vi "BRig_RT__Case_Exp__storeData__endExp__v2.vi"(0 "input_dataBlock":u16[][](array[numeric]), 1 "input_dataCurrent":u16[](array[numeric]), 2 "input_dataLick":u16[][](array[numeric]), 3 "input_dataLC":u16[](array[numeric]), 4 "input_dataExp":u16[](array[numeric]), 5 "input_dataTrial":u16[][](array[numeric]), 7 "input_dataExp_end":u16[](array[numeric]), 9 "input_dataLC_end":u16[](array[numeric]), 11 "input_dataMTrig":u16[](array[numeric]), 12 "input_dataAnalog":u16[][](array[numeric]), 13 "input_dataAnalog_length":i32) -> ()   [LabVIEW 2014]
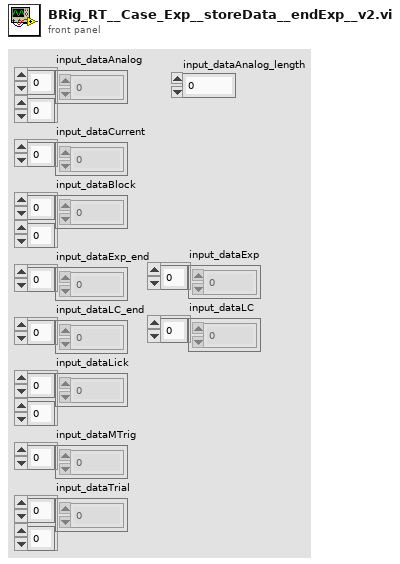
[diagram p1: front panel]
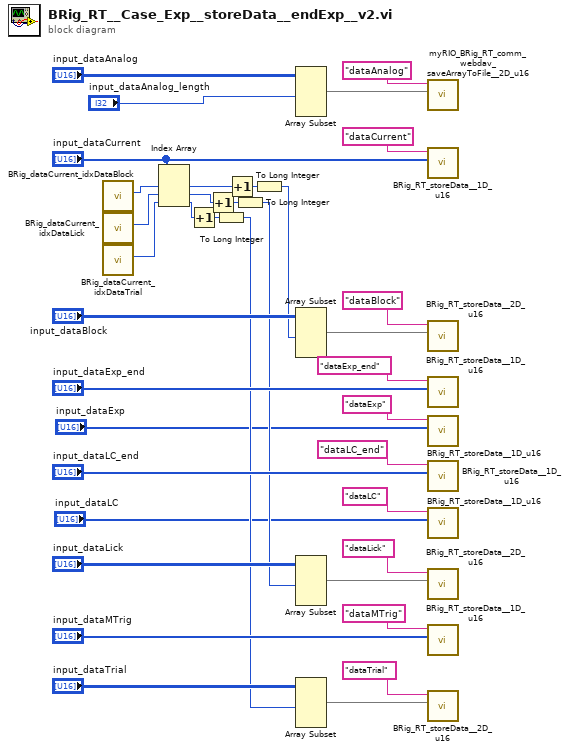
[diagram p0: block diagram]
diagram:
  n1 = call "BRig_dataCurrent_idxDataBlock.vi"() -> ("output_idxDataBlock"=w35:i32)  [unwired: 11 in]
  n2 = call "BRig_dataCurrent_idxDataLick.vi"() -> ("output_idxDataLick"=w34:i32)  [unwired: 11 in]
  n3 = call "BRig_dataCurrent_idxDataTrial.vi"() -> ("output_idxDataTrial"=w33:i32)  [unwired: 11 in]
  n4 = Index Array(array="input_dataCurrent", index #1=w35, index #2=w34, index #3=w33) -> (element #1=w29:u16, element #2=w26:u16, element #3=w23:u16)
  n5 = Increment(x=w23) -> (x+1=w24:u16)
  n6 = Increment(x=w26) -> (x+1=w25:u16)
  n7 = To Long Integer(number=w24) -> (32bit integer=w9:i32)
  n8 = Increment(x=w29) -> (x+1=w28:u16)
  n9 = To Long Integer(number=w25) -> (32bit integer=w15:i32)
  n10 = To Long Integer(number=w28) -> (32bit integer=w27:i32)
  n11 = Array Subset(array="input_dataAnalog", length (row)="input_dataAnalog_length") -> (w7:u16[][])  [unwired: 3 in]
  n12 = Array Subset(array="input_dataBlock", length (row)=w27) -> (w31:u16[][])  [unwired: 3 in]
  n13 = Array Subset(array="input_dataLick", length (row)=w15) -> (w18:u16[][])  [unwired: 3 in]
  n14 = Array Subset(array="input_dataTrial", length (row)=w9) -> (w12:u16[][])  [unwired: 3 in]
  n15 = call "myRIO_BRig_RT_comm_webdav_saveArrayToFile__2D_u16.vi"("Array"=w7, "input_filename"="dataAnalog") -> ()  [unwired: 10 in]
  n16 = call "BRig_RT_storeData__1D_u16.vi"("Array"="input_dataCurrent", "input_filename"="dataCurrent") -> ()  [unwired: 10 in]
  n17 = call "BRig_RT_storeData__2D_u16.vi"("Array"=w31, "input_filename"="dataBlock") -> ()  [unwired: 10 in]
  n18 = call "BRig_RT_storeData__1D_u16.vi"("Array"="input_dataExp_end", "input_filename"="dataExp_end") -> ()  [unwired: 10 in]
  n19 = call "BRig_RT_storeData__1D_u16.vi"("Array"="input_dataExp", "input_filename"="dataExp") -> ()  [unwired: 10 in]
  n20 = call "BRig_RT_storeData__1D_u16.vi"("Array"="input_dataLC_end", "input_filename"="dataLC_end") -> ()  [unwired: 10 in]
  n21 = call "BRig_RT_storeData__1D_u16.vi"("Array"="input_dataLC", "input_filename"="dataLC") -> ()  [unwired: 10 in]
  n22 = call "BRig_RT_storeData__2D_u16.vi"("Array"=w18, "input_filename"="dataLick") -> ()  [unwired: 10 in]
  n23 = call "BRig_RT_storeData__1D_u16.vi"("Array"="input_dataMTrig", "input_filename"="dataMTrig") -> ()  [unwired: 10 in]
  n24 = call "BRig_RT_storeData__2D_u16.vi"("Array"=w12, "input_filename"="dataTrial") -> ()  [unwired: 10 in]
